vi "CAL_GCP_R_power.vi"(9 "Parma In 2":T1, 10 "B_ACC":sgl, 11 "R_ROLL":sgl) -> (0 "R_Period":sgl, 1 "R_GCP":sgl, 2 "R_Ctrl_Start":bool, 3 "R_NUM":u32, 4 "R_Run_OK":bool)   [LabVIEW 2019]
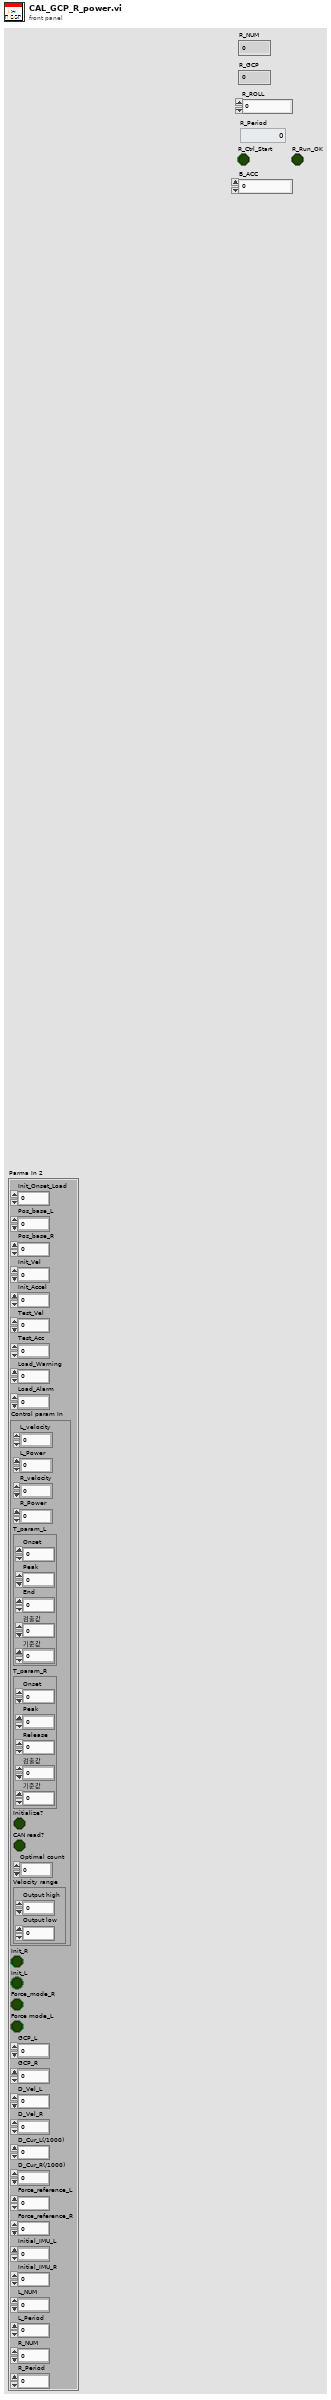
[diagram p1: front panel]
types:
  T1 = cluster{"Init_Onset_Load":sgl, "Pos_base_L":sgl, "Pos_base_R":sgl, "Init_Vel":i32, "Init_Accel":u32, "Test_Vel":i32, "Test_Acc":u32, "Load_Warning":sgl, "Load_Alarm":sgl, "Control param In":cluster{"L_velocity":u32, "L_Power":sgl, "R_velocity":u32, "R_Power":sgl, "T_param_L":cluster{"Onset":sgl, "Peak":sgl, "End":sgl, "검출값":sgl, "기준값":sgl}, "T_param_R":cluster{"Onset":sgl, "Peak":sgl, "Release":sgl, "검출값":sgl, "기준값":sgl}, "Initialize?":bool, "CAN read?":bool, "Optimal count":i32, "Velocity range":cluster{"Output high":dbl, "Output low":dbl}}, "Init_R":bool, "Init_L":bool, "Force_mode_R":bool, "Force mode_L":bool, "GCP_L":sgl, "GCP_R":sgl, "D_Vel_L":sgl, "D_Vel_R":sgl, "D_Cur_L(/1000)":sgl, "D_Cur_R(/1000)":sgl, "Force_reference_L":sgl, "Force_reference_R":sgl, "Initial_IMU_L":sgl, "Initial_IMU_R":sgl, "L_NUM":u32, "L_Period":i16, "R_NUM":u32, "R_Period":i16}
  T2 = enum16{"Init", "HF", "Cross", "HE", "Cross_E", "Init_F"}
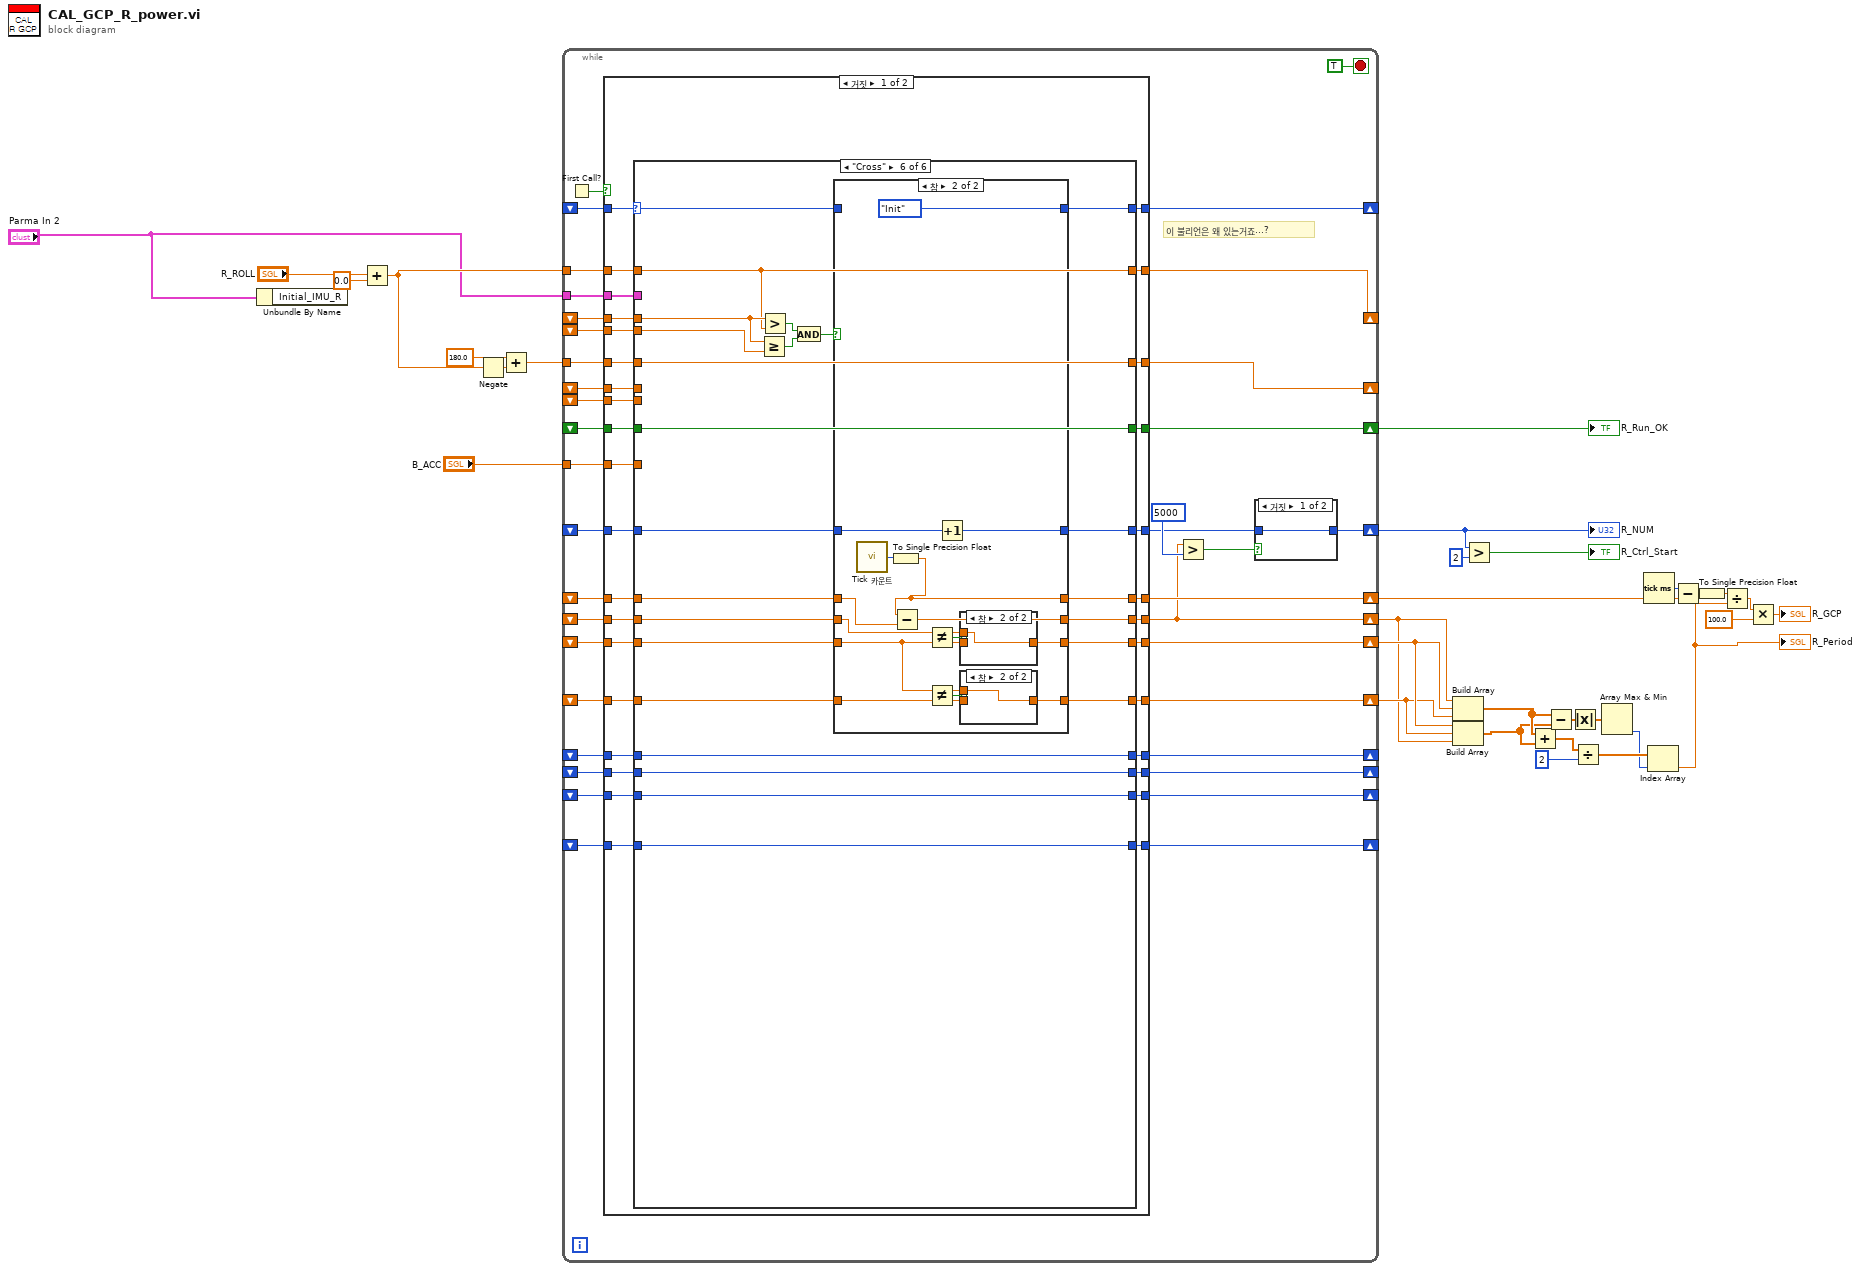
[diagram p0: block diagram]
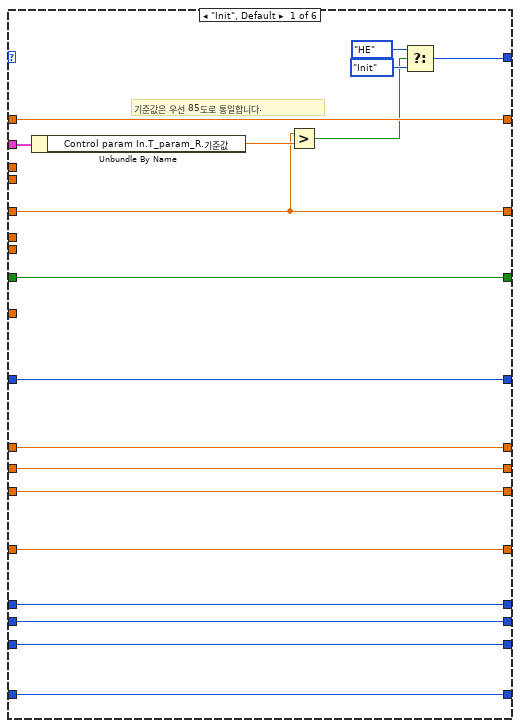
[diagram p2: hidden frame]
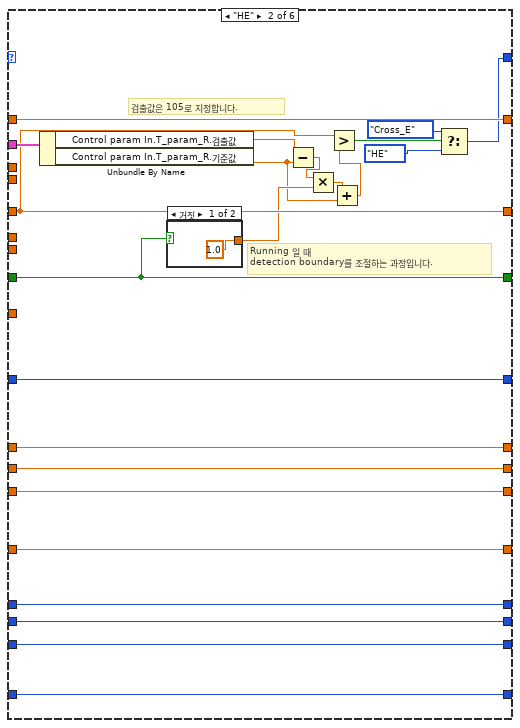
[diagram p3: hidden frame]
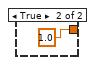
[diagram p4: hidden frame]
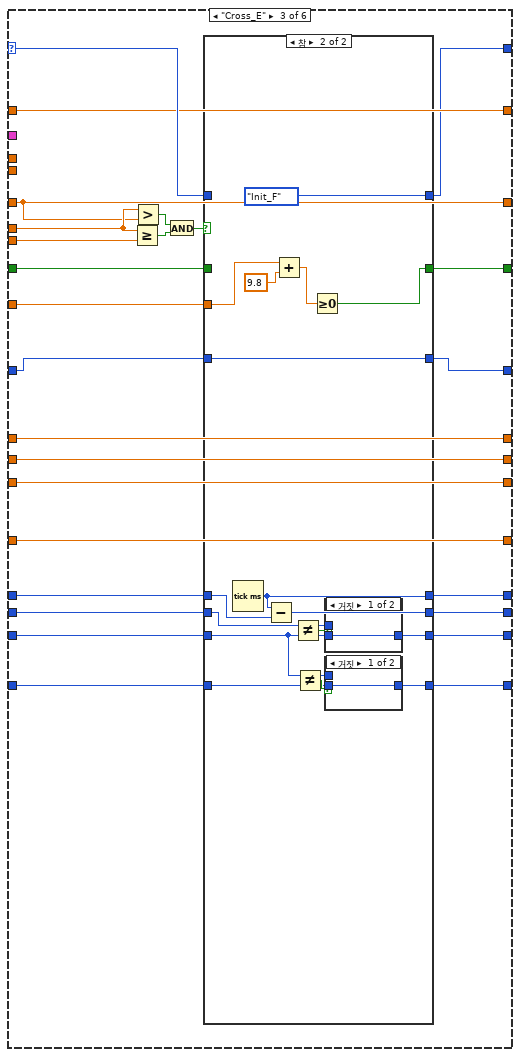
[diagram p5: hidden frame]
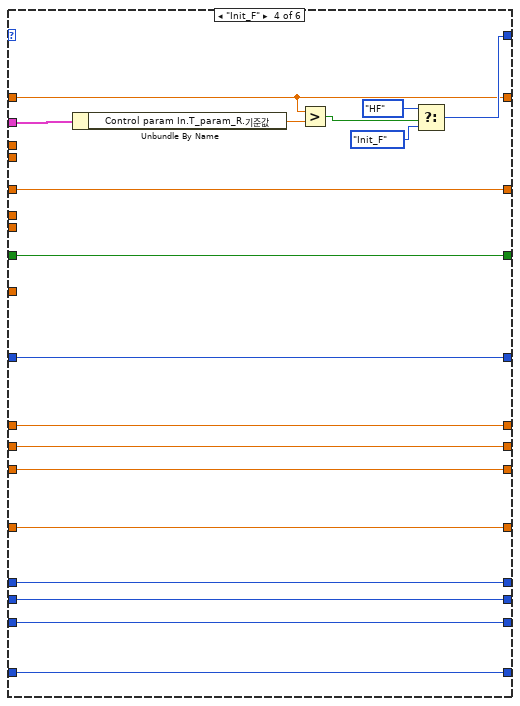
[diagram p9: hidden frame]
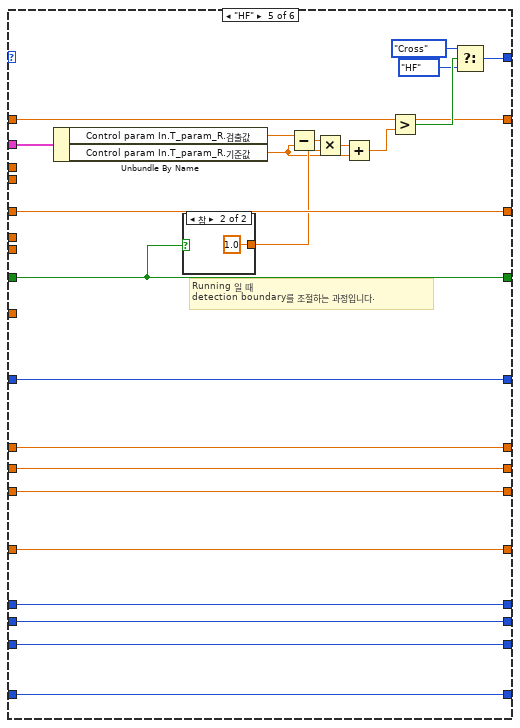
[diagram p10: hidden frame]
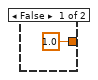
[diagram p11: hidden frame]
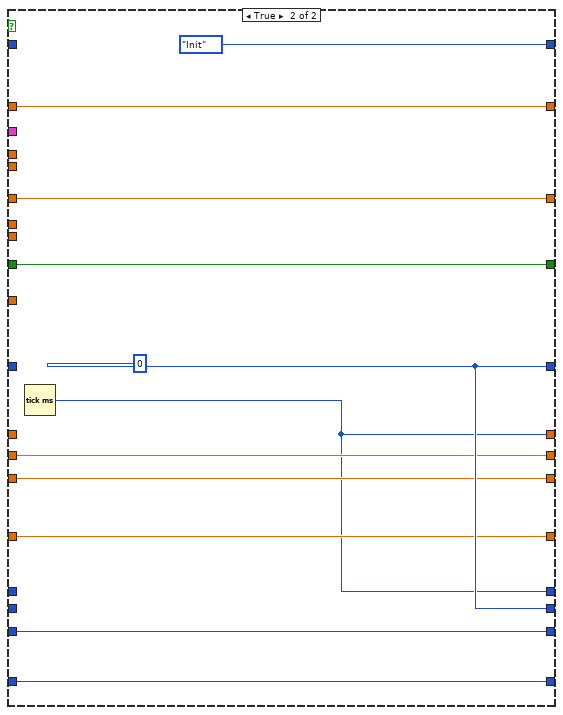
[diagram p15: hidden frame]
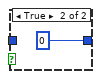
[diagram p16: hidden frame]
diagram:
  n1 = Unbundle By Name("Parma In 2") -> ()  [unwired: 1 out]
  n2 = Add(x="R_ROLL", y=sgl 0.0) -> (x+y=w3:sgl)
  n3 = Negate(x=w3) -> (-x=w23:sgl)
  n4 = Add(x=sgl 180.0, y=w23) -> (x+y=w20:sgl)
  n5 = while {
    tunnel: w3 -> [w65]
    tunnel: "Parma In 2" -> [w62]
    shift-right: [w34] -> _
    shift-left: _ -> [w33]
    shift-right: [w66] -> _
    shift-left: _ -> [w61]
    shift-left: _ -> [w60]
    shift-right: [w57] -> w18
    shift-left: _ -> [w64]
    shift-right: [w47] -> _
    shift-left: _ -> [w63]
    tunnel: w20 -> [w55]
    shift-right: [w54] -> _
    shift-left: _ -> [w53]
    shift-left: _ -> [w52]
    shift-right: [w51] -> w19
    shift-left: _ -> [w50]
    tunnel: "B_ACC" -> [w49]
    shift-right: [w46] -> _
    shift-left: _ -> [w48]
    shift-right: [w39] -> w11
    shift-left: _ -> [w38]
    shift-right: [w36] -> w10
    shift-left: _ -> [w37]
    shift-right: [w45] -> _
    shift-left: _ -> [w44]
    shift-right: [w42] -> _
    shift-left: _ -> [w43]
    shift-right: [w41] -> w17
    shift-left: _ -> [w40]
    shift-right: [w32] -> w9
    shift-left: _ -> [w35]
    stop <- TRUE stop-if-true
    # "이 불리언은 왜 있는거죠...?"
    n6 = First Call?() -> (First Call?: T/F=w67:bool)
    n7 = case shown="거짓" w67 {
      tunnel: [w98 w298] -> w66
      tunnel: w65 -> [w99 w298]
      tunnel: w64 -> [w96 _]
      tunnel: [w97 w297] -> w56
      tunnel: [w94 w288] -> w47
      tunnel: [w93 w297] -> w46
      tunnel: w63 -> [w95 _]
      tunnel: w62 -> [w100 _]
      tunnel: w61 -> [w92 _]
      tunnel: w60 -> [w91 _]
      tunnel: w55 -> [w90 w296]
      tunnel: [w89 w296] -> w54
      tunnel: w53 -> [w88 _]
      tunnel: w52 -> [w87 _]
      tunnel: [w85 w295] -> w51
      tunnel: w50 -> [w86 w295]
      tunnel: w49 -> [w84 _]
      tunnel: w48 -> [w83 _]
      tunnel: [w82 w294] -> w45
      tunnel: w44 -> [w81 w294]
      tunnel: w43 -> [w80 w293]
      tunnel: [w79 w293] -> w42
      tunnel: [w78 w288] -> w41
      tunnel: w40 -> [w77 _]
      tunnel: [w76 w292] -> w39
      tunnel: w38 -> [w75 w292]
      tunnel: w37 -> [w74 w291]
      tunnel: [w73 w291] -> w36
      tunnel: [w72 w290] -> w32
      tunnel: w35 -> [w71 w290]
      tunnel: [w69 T2."Init"] -> w34
      tunnel: w33 -> [w70 _]
      frame False {
        n8 = case shown="\"Cross\"" w70 {
          selector: w70 -> [_ _ w169 _ _ w263]
          tunnel: w100 -> [w117 w133 _ w211 w237 _]
          tunnel: w99 -> [w116 w140 w151 w209 w235 w256]
          tunnel: [w116 w140 w151 w209 w235 w256] -> w98
          tunnel: [w115 w139 w167 w206 w234 w258] -> w97
          tunnel: w96 -> [w115 w139 w168 w206 w234 w259]
          tunnel: w95 -> [w114 w138 w165 w205 w233 w251]
          tunnel: [w114 w138 w166 w205 w233 w251] -> w94
          tunnel: [w111 w137 w164 w204 w232 w254] -> w93
          tunnel: w92 -> [_ _ _ _ _ w257]
          tunnel: w91 -> [_ _ _ _ _ w262]
          tunnel: w90 -> [w113 w132 w150 w208 w228 w248]
          tunnel: [w113 w132 w150 w208 w228 w248] -> w89
          tunnel: w88 -> [_ _ w156 _ _ _]
          tunnel: w87 -> [_ _ w157 _ _ _]
          tunnel: w86 -> [w112 w123 w163 w207 w222 w247]
          tunnel: [w112 w123 w162 w207 w222 w247] -> w85
          tunnel: w84 -> [_ _ w161 _ _ _]
          tunnel: w83 -> [w111 w137 w145 w204 w232 w254]
          tunnel: [w110 w136 w155 w202 w231 w253] -> w82
          tunnel: w81 -> [w110 w136 w144 w202 w231 w253]
          tunnel: w80 -> [w109 w135 w154 w201 w230 w252]
          tunnel: [w109 w135 w153 w201 w230 w252] -> w79
          tunnel: [w108 w134 w152 w203 w229 w250] -> w78
          tunnel: w77 -> [w108 w134 w152 w203 w229 w249]
          tunnel: [w107 w131 w148 w199 w227 w246] -> w76
          tunnel: w75 -> [w107 w131 w148 w199 w227 w245]
          tunnel: w74 -> [w106 w130 w149 w198 w226 w244]
          tunnel: [w106 w130 w149 w198 w226 w243] -> w73
          tunnel: [w105 w122 w147 w200 w218 w242] -> w72
          tunnel: w71 -> [w105 w122 w147 w200 w218 w241]
          tunnel: [w104 w119 w146 w210 w215 w240] -> w69
          frame "Init", Default {
            # "기준값은 우선 85도로 통일합니다."
            n9 = Unbundle By Name(w117) -> ("Control param In.T_param_R.기준값"=w118:sgl)
            n10 = Greater?(x=w113, y=w118) -> (0:w101:bool)
            n11 = Select(t=T2."HE", s=w101, f=T2."Init") -> (s? t:f=w104:T2)
          }
          frame "HE" {
            # "Running 일 때 \ndetection boundary를 조절하는 과정입니다."
            # "검출값은 105로 지정합니다."
            n12 = Unbundle By Name(w133) -> ("Control param In.T_param_R.검출값"=w128:sgl, "Control param In.T_param_R.기준값"=w125:sgl)
            n13 = case shown="거짓" w123 {
              tunnel: [sgl 1.0 ("y") sgl 1.0 ("y")] -> w129
              frame False {
              }
              frame True {
              }
            }
            n14 = Subtract(x=w128, y=w125) -> (x-y=w127:sgl)
            n15 = Multiply(x=w127, y=w129) -> (x*y=w126:sgl)
            n16 = Add(x=w126, y=w125) -> (x+y=w124:sgl)
            n17 = Greater?(x=w132, y=w124) -> (0:w141:bool)
            n18 = Select(t=T2."Cross_E", s=w141, f=T2."HE") -> (s? t:f=w119:T2)
          }
          frame "Cross_E" {
            n19 = Greater Or Equal?(x=w156, y=w157) -> (x >= y?=w160:bool)
            n20 = Greater?(x=w156, y=w150) -> (0:w159:bool)
            n21 = And(x=w159, y=w160) -> (x .and. y?=w158:bool)
            n22 = case shown="참" w158 {
              tunnel: w169 -> [w174 _]
              tunnel: [w174 T2."Init_F"] -> w146
              tunnel: w168 -> [w175 w183]
              tunnel: [w175 w183] -> w167
              tunnel: w165 -> [w176 w192]
              tunnel: [w171 w182] -> w164
              tunnel: [w176 w191] -> w166
              tunnel: w163 -> [w173 _]
              tunnel: [w173 w188] -> w162
              tunnel: w161 -> [_ w177]
              tunnel: [w170 w187] -> w155
              tunnel: w154 -> [w172 w186]
              tunnel: [w172 w185] -> w153
              tunnel: w145 -> [w171 w181]
              tunnel: w144 -> [w170 w180]
              frame False {
              }
              frame True {
                n23 = Tick Count (ms)() -> (millisecond timer value=w191:u32)
                n24 = Subtract(x=w191, y=w192) -> (x-y=w182:u32)
                n25 = Add(x=w177, y=9.8) -> (x+y=w178:dbl)
                n26 = Not Equal?(x=w181, y=w180) -> (x != y?=w190:bool)
                n27 = Not Equal?(x=w180, y=w186) -> (x != y?=w189:bool)
                n28 = Greater Or Equal To 0?(x=w178) -> (x >= 0?=w188:bool)
                n29 = case shown="거짓" w190 {
                  tunnel: [w195 w196] -> w187
                  tunnel: w181 -> [_ w196]
                  tunnel: w180 -> [w195 _]
                  frame False {
                  }
                  frame True {
                  }
                }
                n30 = case shown="거짓" w189 {
                  tunnel: w180 -> [_ w194]
                  tunnel: w186 -> [w193 _]
                  tunnel: [w193 w194] -> w185
                  frame False {
                  }
                  frame True {
                  }
                }
              }
            }
          }
          frame "Init_F" {
            n31 = Unbundle By Name(w211) -> ("Control param In.T_param_R.기준값"=w214:sgl)
            n32 = Greater?(x=w209, y=w214) -> (0:w197:bool)
            n33 = Select(t=T2."HF", s=w197, f=T2."Init_F") -> (s? t:f=w210:T2)
          }
          frame "HF" {
            # "Running 일 때 \ndetection boundary를 조절하는 과정입니다."
            n34 = Unbundle By Name(w237) -> ("Control param In.T_param_R.검출값"=w225:sgl, "Control param In.T_param_R.기준값"=w220:sgl)
            n35 = case shown="참" w222 {
              tunnel: [sgl 1.0 ("y") sgl 1.0 ("y")] -> w223
              frame False {
              }
              frame True {
              }
            }
            n36 = Subtract(x=w225, y=w220) -> (x-y=w224:sgl)
            n37 = Multiply(x=w224, y=w223) -> (x*y=w221:sgl)
            n38 = Add(x=w221, y=w220) -> (x+y=w219:sgl)
            n39 = Greater?(x=w235, y=w219) -> (0:w236:bool)
            n40 = Select(t=T2."Cross", s=w236, f=T2."HF") -> (s? t:f=w215:T2)
          }
          frame "Cross" {
            n41 = Greater Or Equal?(x=w257, y=w262) -> (x >= y?=w261:bool)
            n42 = Greater?(x=w257, y=w256) -> (0:w255:bool)
            n43 = And(x=w255, y=w261) -> (x .and. y?=w260:bool)
            n44 = case shown="참" w260 {
              tunnel: w263 -> [w268 _]
              tunnel: [w268 T2."Init"] -> w240
              tunnel: w259 -> [w269 w275]
              tunnel: [w269 w274] -> w258
              tunnel: [w267 w270] -> w250
              tunnel: w249 -> [w267 w281]
              tunnel: [w266 w280] -> w246
              tunnel: w245 -> [w266 w272]
              tunnel: w244 -> [w265 w279]
              tunnel: [w265 w278] -> w243
              tunnel: [w264 w277] -> w242
              tunnel: w241 -> [w264 w273]
              frame False {
              }
              frame True {
                n45 = call "Tick 카운트"() -> ("Tick Count(mSec)"=w271:u32)
                n46 = To Single Precision Float(number=w271) -> (single precision float=w270:sgl)
                n47 = Subtract(x=w270, y=w281) -> (x-y=w277:sgl)
                n48 = Not Equal?(x=w273, y=w272) -> (x != y?=w283:bool)
                n49 = Not Equal?(x=w272, y=w279) -> (x != y?=w282:bool)
                n50 = Increment(x=w275) -> (x+1=w274:u32)
                n51 = case shown="참" w283 {
                  tunnel: w273 -> [_ w287]
                  tunnel: [w286 w287] -> w280
                  tunnel: w272 -> [w286 _]
                  frame False {
                  }
                  frame True {
                  }
                }
                n52 = case shown="참" w282 {
                  tunnel: w272 -> [_ w285]
                  tunnel: w279 -> [w284 _]
                  tunnel: [w284 w285] -> w278
                  frame False {
                  }
                  frame True {
                  }
                }
              }
            }
          }
        }
      }
      frame True {
        w297 = u32 0
        n53 = Tick Count (ms)() -> (millisecond timer value=w288:u32)
      }
    }
    n54 = Greater?(x=w32, y=u32 5000) -> (0:w58:bool)
    n55 = case shown="거짓" w58 {
      tunnel: [w299 u32 0] -> w57
      tunnel: w56 -> [w299 _]
      frame False {
      }
      frame True {
      }
    }
  }
  "R_NUM" <- w18
  "R_Run_OK" <- w19
  n56 = Build Array(w9, w11, w10) -> (w7:sgl[])
  n57 = Build Array(w11, w10, w9) -> (w6:sgl[])
  n58 = Greater?(x=w18, y=u32 2) -> (0:→"R_Ctrl_Start":bool)
  n59 = Add(x=w7, y=w6) -> (x+y=w14:sgl[])
  n60 = Subtract ("빼기")(x=w7, y=w6) -> (x-y=w16:sgl[])
  n61 = Absolute Value(x=w16) -> (abs(x)=w15:sgl[])
  n62 = Divide ("나누기")(x=w14, y=2) -> (x/y=w12:sgl[])
  n63 = Array Max & Min(array=w15) -> (min index (indices)=w5:i32)  [unwired: 3 out]
  n64 = Tick Count (ms)() -> (millisecond timer value=w27:u32)
  n65 = Index Array(array=w12, index=w5) -> (element=w8:sgl)
  "R_Period" <- w8
  n66 = Subtract(x=w27, y=w17) -> (x-y=w26:sgl)
  n67 = To Single Precision Float(number=w26) -> (single precision float=w22:sgl)
  n68 = Divide(x=w22, y=w8) -> (x/y=w29:sgl)
  n69 = Multiply(x=w29, y=sgl 100.0) -> (x*y=→"R_GCP":sgl)
